vi "B_sweep_versus time_3ch_DR_v2.1.vi"(1 "name or relative path":string="Bsweeps_lockin_sweepVsg1&Vsg2_Vbg9V", 3 "description":string="SA02610M.20130217\ntemp=100mK\n1mVac+350uVdc\nVbg=1V\n", 5 "Stop":bool, 8 "slow scan through zero?":bool, 11 "sec to stablize B":u32=10, 15 "B Start (Oe)":dbl=20000.0, 16 "B End (Oe)":dbl=-20000.0, 17 "B Scan (Oe/sec)":dbl=10.0) -> (0 "Pickering":string="Vbg:27\nV1+:2\nI-:4\nI+:1\nV2-:5\nV2-:28\nV2+:2\nV-:3\n", 10 "Zx 2":cluster{"Y":dbl[], "Y":dbl[]}(graph), 12 "Zx":cluster{"Y":dbl[], "Y":dbl[]}(graph), 13 "T":cluster{"Y":dbl[], "Y":dbl[]}(graph), 18 "Y Channel":cluster{"Y":dbl[], "Y":dbl[]}(graph), 19 "X Channel":cluster{"Y":dbl[], "Y":dbl[]}(graph))   [LabVIEW 2011]
uses:
  SubVI/ITX_Global.vi
  DAQ-lockin-SubVI/Source/Lock-in Globles.vi
panel:
  out "Current field (Oe)":dbl=-19995.404
  in  "Tab Control":T1(tab)
  in  "Lock-in #":u16(ring) items=["Lock-in #1", "Lock-in #2", "Lock-in #3", "Lock-in #4"]
  in  "Lock-in # 3":u16(ring)=2 items=["Lock-in #1", "Lock-in #2", "Lock-in #3", "Lock-in #4"]
  in  "Lock-in # 4":u16(ring)=3 items=["Lock-in #1", "Lock-in #2", "Lock-in #3", "Lock-in #4"]
  in  "Device image":path=path "C:/Experiments/2011-summer Superconductivity-Spin Hall/Device images/SA02610M.20121218.png"
  out "Last Scan Image":T2(plugin-control)
  in  "Initial Rate (Oe/s)":i32=100
  in  "Stop Lockin":bool
  out "X 3":cluster{"Y":dbl[], "Y":dbl[]}(graph)
  out "Y 3":cluster{"Y":dbl[], "Y":dbl[]}(graph)
  out "X 4":cluster{"Y":dbl[], "Y":dbl[]}(graph)
  out "Y4":cluster{"Y":dbl[], "Y":dbl[]}(graph)
  out "Zy":cluster{"Y":dbl[], "Y":dbl[]}(graph)
  out "Zy 2":cluster{"Y":dbl[], "Y":dbl[]}(graph)
  out "T 2":cluster{"Y":dbl[], "Y":dbl[]}[](graph)
  # "yes"
  # "no"
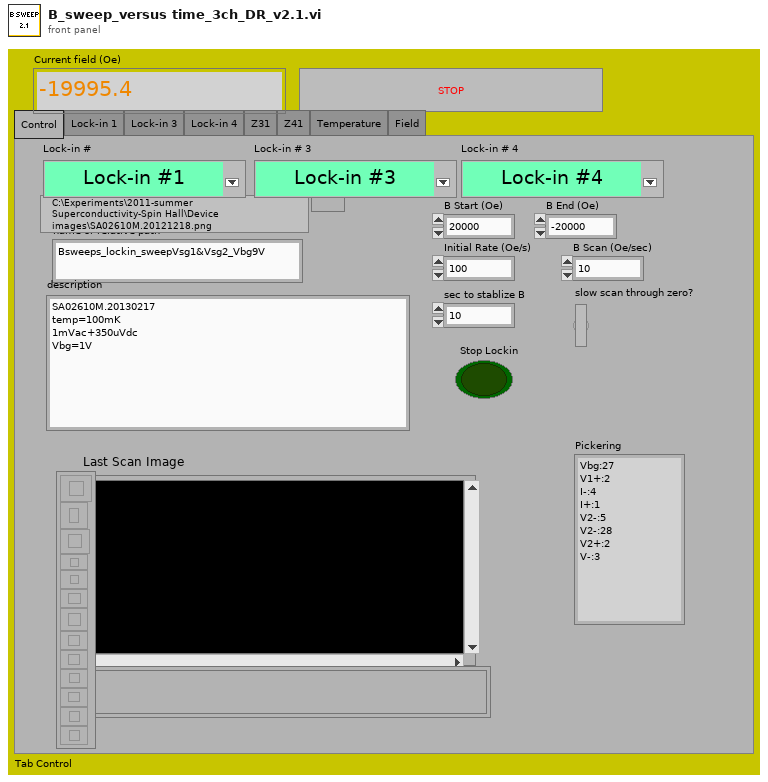
[diagram p1: front panel]
types:
  T1 = enum32{"Control", "Lock-in 1", "Lock-in 3", "Lock-in 4", "Z31", "Z41", "Temperature", "Field"}
  T2 = typedef "IMAQ Image.ctl" = refnum<image>
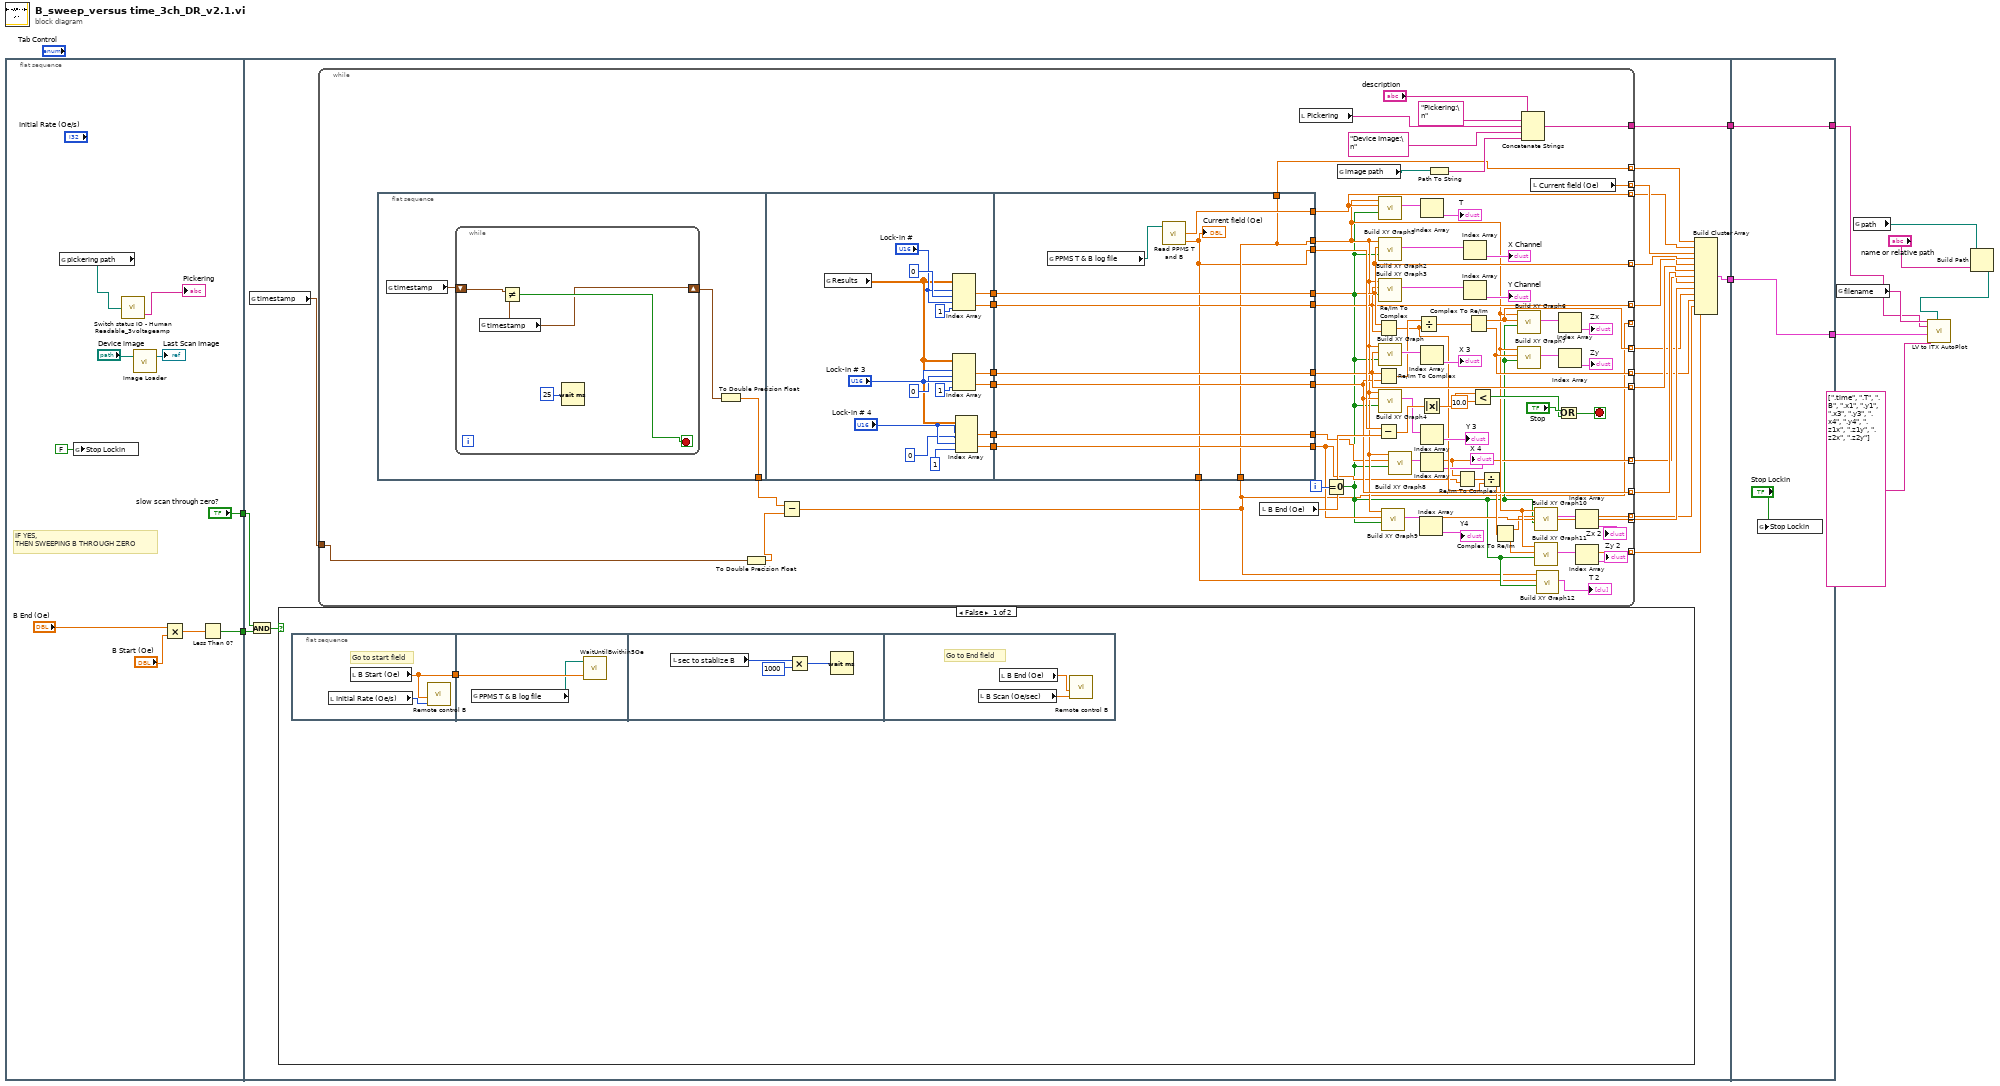
[diagram p0: block diagram]
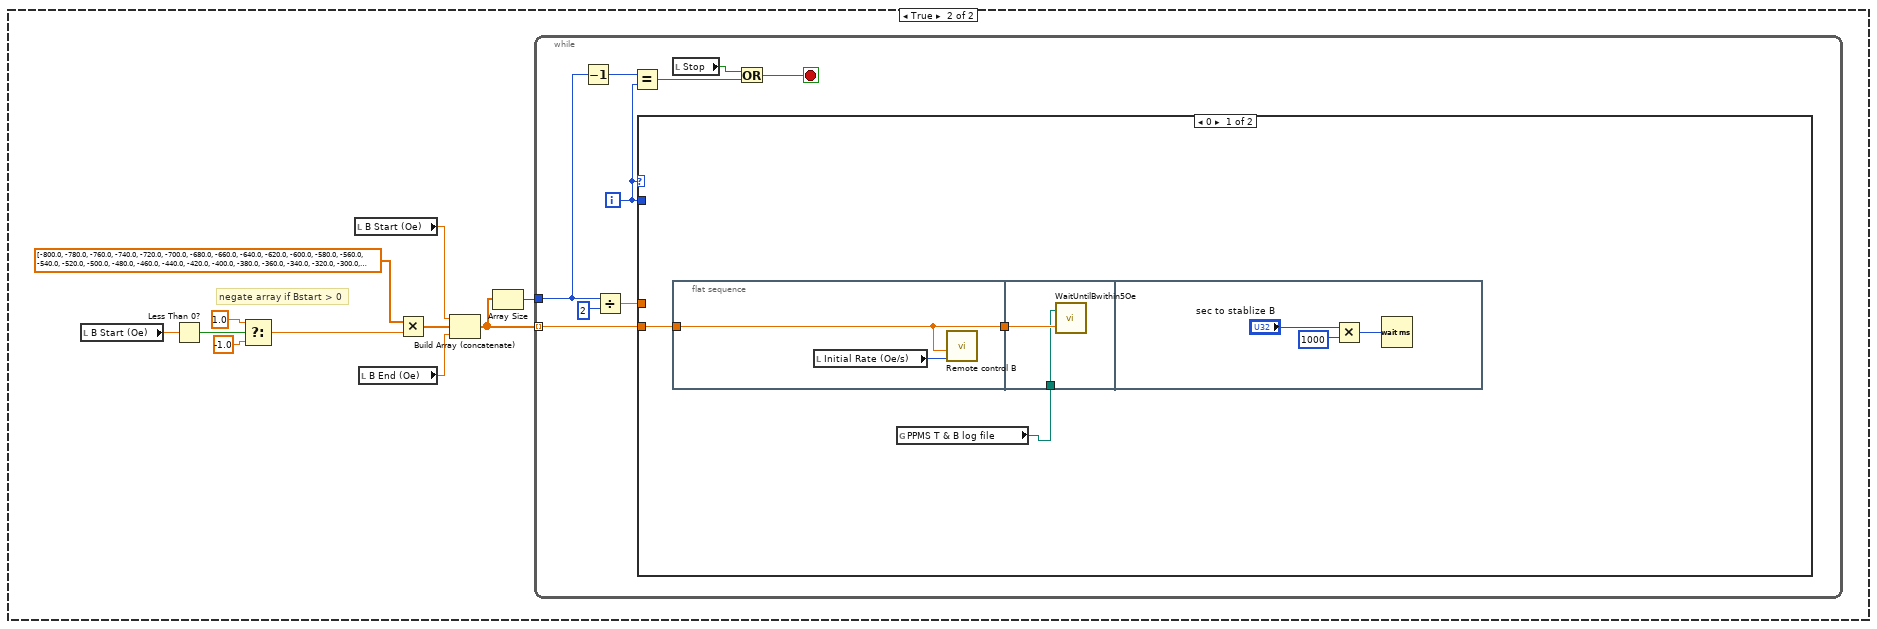
[diagram p2: hidden frame]
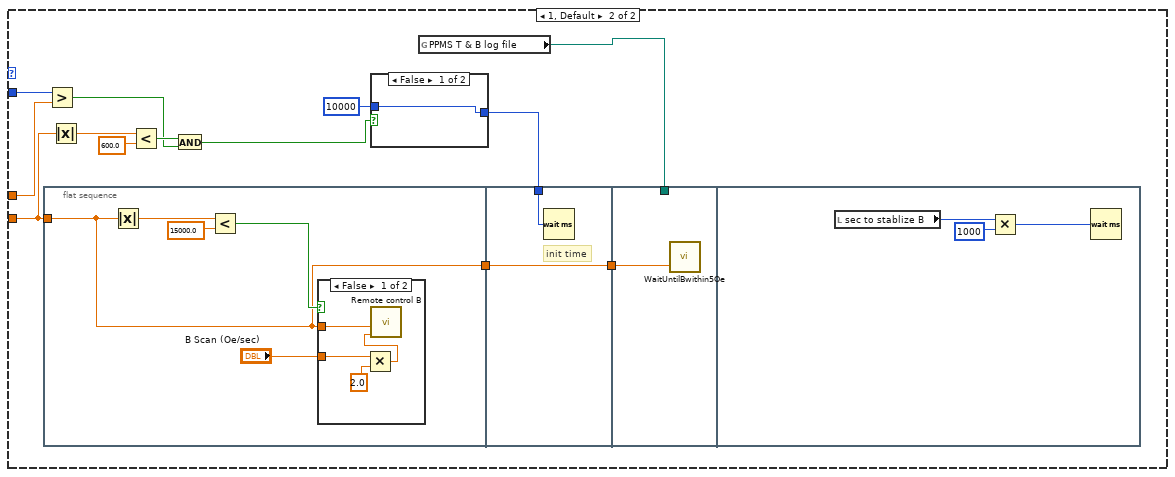
[diagram p3: hidden frame]
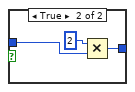
[diagram p4: hidden frame]
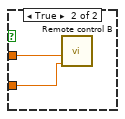
[diagram p5: hidden frame]
diagram:
  n1 = flat-sequence {
    tunnel: [w20] -> w11
    tunnel: ["slow scan through zero?"] -> w10
    tunnel: w11 -> [w40]
    tunnel: w10 -> [w39]
    tunnel: [w37] -> w7
    tunnel: [w24] -> w2
    tunnel: [w220] -> w4
    tunnel: w7 -> [w220]
    tunnel: [w218] -> w3
    tunnel: w2 -> [w218]
    frame #0 {
      # "IF YES,\nTHEN SWEEPING B THROUGH ZERO"
      n2 = global read "ITX_Global.vi" "pickering path"() -> (w13:path)
      n3 = global write "Lock-in Globles.vi" "Stop Lockin"(FALSE ("Stop Lockin")) -> ()
      n4 = call <userlib>:"Switch status IO - Human Readable_3voltageamp.vi"("Switch status"=w13) -> ("String"=→"Pickering":string)  [unwired: 3 in]
      n5 = call "Image Loader.vi"("File Path"="Device image") -> ("Last Scan Image"=→"Last Scan Image":T2)  [unwired: 2 in]
      n6 = Multiply(x="B End (Oe)", y="B Start (Oe)") -> (x*y=w21:dbl)
      n7 = Less Than 0?(x=w21) -> (x < 0?=w20:bool)
    }
    frame #1 {
      n8 = global read "Lock-in Globles.vi" "timestamp"() -> (w22:timestamp)
      n9 = And(x=w39, y=w40) -> (x .and. y?=w38:bool)
      n10 = case shown="False" w38 {
        frame False {
          n11 = flat-sequence {
            tunnel: [w42] -> w41
            tunnel: w41 -> [w45]
            frame #0 {
              # "Go to start field"
              n12 = local read "Initial Rate (Oe/s)"() -> (w43:i32)
              n13 = local read "B Start (Oe)"() -> (w42:dbl)
              n14 = call "Remote control B.vi"("Rate (Oe/s)"=w43, "Field (Oe)"=w42) -> ()  [unwired: 7 in, 1 out]
            }
            frame #1 {
              n15 = global read "ITX_Global.vi" "PPMS T & B log file"() -> (w44:path)
              n16 = call "WaitUntilBwithin5Oe.vi"("Target Field (Oe)"=w45, "PPMS T & B log file"=w44) -> ()  [unwired: 2 in]
            }
            frame #2 {
              n17 = local read "sec to stablize B"() -> (w46:u32)
              n18 = Multiply(x=w46, y=u32 1000) -> (x*y=w47:u32)
              n19 = Wait (ms)(milliseconds to wait=w47) -> ()  [unwired: 1 out]
            }
            frame #3 {
              # "Go to End field"
              n20 = local read "B Scan (Oe/sec)"() -> (w49:dbl)
              n21 = local read "B End (Oe)"() -> (w50:dbl)
              n22 = call "Remote control B.vi"("Rate (Oe/s)"=w49, "Field (Oe)"=w50) -> ()  [unwired: 7 in, 1 out]
            }
          }
        }
        frame True {
          # "negate array if Bstart > 0"
          n23 = local read "B Start (Oe)"() -> (w61:dbl)
          n24 = Less Than 0?(x=w61) -> (x < 0?=w59:bool)
          n25 = Select(t=1.0, s=w59, f=-1.0) -> (s? t:f=w58:dbl)
          n26 = local read "B Start (Oe)"() -> (w53:dbl)
          n27 = local read "B End (Oe)"() -> (w54:dbl)
          n28 = Multiply(x=dbl[] [-800.0, -780.0, -760.0, -740.0, -720.0, -700.0, -680.0, -660.0, -640.0, -620.0, -600.0, -580.0, -560.0, -540.0, -520.0, -500.0, -480.0, -460.0, -440.0, -420.0, -400.0, -380.0, -360.0, -340.0, -320.0, -300.0, -280.0, -260.0, -240.0, -220.0, -200.0, -190.0, -180.0, -170.0, -160.0, -150.0, -140.0, -130.0, -120.0, -110.0, -100.0, -90.0, -80.0, -70.0, -60.0, -50.0, -40.0, -30.0, -20.0, -10.0, 0.0, 10.0, 20.0, 30.0, 40.0, 50.0, 60.0, 70.0, 80.0, 90.0, 100.0, 110.0, 120.0, 130.0, 140.0, 150.0, 160.0, 170.0, 180.0, 190.0, 200.0, 220.0, 240.0, 260.0, 280.0, 300.0, 320.0, 340.0, 360.0, 380.0, 400.0, 420.0, 440.0, 460.0, 480.0, 500.0, 520.0, 540.0, 560.0, 580.0, 600.0, 620.0, 640.0, 660.0, 680.0, 700.0, 720.0, 740.0, 760.0, 780.0, 800.0], y=w58) -> (x*y=w55:dbl[])
          n29 = Build Array (concatenate)(w53, w55, w54) -> (w52:dbl[])
          n30 = Array Size(array=w52) -> (size(s)=w51:i32)
          n31 = while {
            tunnel: w52 -> [w70] mode=indexing
            tunnel: w51 -> [w65]
            i -> [w62]
            stop <- w66 stop-if-true
            n32 = Decrement(x=w65) -> (x-1=w69:i32)
            n33 = Divide(x=w65, y=2) -> (x/y=w63:dbl)
            n34 = Equal?(x=w69, y=w62) -> (x = y?=w68:bool)
            n35 = case shown="0" w62 {
              tunnel: w70 -> [w72 w91]
              tunnel: w63 -> [_ w87]
              tunnel: w62 -> [_ w86]
              frame 0 {
                n36 = flat-sequence {
                  tunnel: w72 -> [w75]
                  tunnel: [w75] -> w73
                  tunnel: w71 -> [w76]
                  tunnel: w73 -> [w77]
                  frame #0 {
                    n37 = local read "Initial Rate (Oe/s)"() -> (w74:i32)
                    n38 = call "Remote control B.vi"("Rate (Oe/s)"=w74, "Field (Oe)"=w75) -> ()  [unwired: 7 in, 1 out]
                  }
                  frame #1 {
                    n39 = call "WaitUntilBwithin5Oe.vi"("Target Field (Oe)"=w77, "PPMS T & B log file"=w76) -> ()  [unwired: 2 in]
                  }
                  frame #2 {
                    n40 = Multiply(x="sec to stablize B", y=u32 1000) -> (x*y=w79:u32)
                    n41 = Wait (ms)(milliseconds to wait=w79) -> ()  [unwired: 1 out]
                  }
                }
                n42 = global read "ITX_Global.vi" "PPMS T & B log file"() -> (w71:path)
              }
              frame 1, Default {
                n43 = flat-sequence {
                  tunnel: w91 -> [w99]
                  tunnel: [w99] -> w93
                  tunnel: w93 -> [w110]
                  tunnel: [w110] -> w92
                  tunnel: w82 -> [w109]
                  tunnel: w81 -> [_]
                  tunnel: w92 -> [w111]
                  frame #0 {
                    n44 = Absolute Value(x=w99) -> (abs(x)=w98:dbl)
                    n45 = Less?(x=w98, y=15000.0) -> (x < y?=w100:bool)
                    n46 = case shown="False" w100 {
                      tunnel: w99 -> [w106 w108]
                      tunnel: "B Scan (Oe/sec)" -> [w105 w107]
                      frame False {
                        n47 = Multiply(x=w105, y=2.0) -> (x*y=w103:dbl)
                        n48 = call "Remote control B.vi"("Rate (Oe/s)"=w103, "Field (Oe)"=w106) -> ()  [unwired: 7 in, 1 out]
                      }
                      frame True {
                        n49 = call "Remote control B.vi"("Rate (Oe/s)"=w107, "Field (Oe)"=w108) -> ()  [unwired: 7 in, 1 out]
                      }
                    }
                  }
                  frame #1 {
                    # "init time"
                    n50 = Wait (ms)(milliseconds to wait=w109) -> ()  [unwired: 1 out]
                  }
                  frame #2 {
                    n51 = call "WaitUntilBwithin5Oe.vi"("Target Field (Oe)"=w111) -> ()  [unwired: 3 in]
                  }
                  frame #3 {
                    n52 = local read "sec to stablize B"() -> (w112:u32)
                    n53 = Multiply(x=w112, y=u32 1000) -> (x*y=w113:u32)
                    n54 = Wait (ms)(milliseconds to wait=w113) -> ()  [unwired: 1 out]
                  }
                }
                n55 = Greater?(x=w86, y=w87) -> (0:w85:bool)
                n56 = Absolute Value(x=w91) -> (abs(x)=w88:dbl)
                n57 = Less?(x=w88, y=600.0) -> (x < y?=w89:bool)
                n58 = And(x=w89, y=w85) -> (x .and. y?=w84:bool)
                n59 = case shown="False" w84 {
                  tunnel: u32 10000 ("y") -> [w94 w97]
                  tunnel: [w94 w95] -> w82
                  frame False {
                  }
                  frame True {
                    n60 = Multiply(x=u32 2, y=w97) -> (x*y=w95:u32)
                  }
                }
                n61 = global read "ITX_Global.vi" "PPMS T & B log file"() -> (w81:path)
              }
            }
            n62 = local read "Stop"() -> (w67:bool)
            n63 = Or(x=w67, y=w68) -> (x .or. y?=w66:bool)
          }
        }
      }
      n64 = while {
        tunnel: [w115] -> _ mode=indexing
        tunnel: [w155] -> w35 mode=indexing
        tunnel: [w154] -> w36 mode=indexing
        tunnel: [w153] -> w34 mode=indexing
        tunnel: [w152] -> w32 mode=indexing
        tunnel: [w151] -> w33 mode=indexing
        tunnel: [w150] -> w31 mode=indexing
        tunnel: [w149] -> w28 mode=indexing
        tunnel: [w148] -> w27 mode=indexing
        tunnel: [w127] -> w37
        tunnel: [w126] -> w30 mode=indexing
        tunnel: [w125] -> w29 mode=indexing
        tunnel: [w124] -> w26 mode=indexing
        tunnel: [w123] -> w25 mode=indexing
        tunnel: [w119] -> w23 mode=indexing
        tunnel: w22 -> [w118]
        i -> [w184]
        stop <- w177 stop-if-true
        n65 = flat-sequence {
          tunnel: [w187] -> w117
          tunnel: [w204] -> w159
          tunnel: [w203] -> w158
          tunnel: [w199] -> w157
          tunnel: [w198] -> w156
          tunnel: [w193] -> w147
          tunnel: [w192] -> w146
          tunnel: [w209] -> w136
          tunnel: [w208] -> w167
          tunnel: w159 -> [w217]
          tunnel: [w217] -> w151
          tunnel: w158 -> [w216]
          tunnel: [w216] -> w153
          tunnel: [w215] -> w152
          tunnel: w157 -> [w215]
          tunnel: w156 -> [w214]
          tunnel: [w214] -> w150
          tunnel: [w213] -> w155
          tunnel: [w212] -> w126
          tunnel: w147 -> [w212]
          tunnel: [w211] -> w125
          tunnel: w146 -> [w211]
          tunnel: w115 -> [w209]
          tunnel: [w208] -> w121
          tunnel: [w209] -> w119
          frame #0 {
            n66 = global read "Lock-in Globles.vi" "timestamp"() -> (w186:timestamp)
            n67 = while {
              shift-right: [w189] -> w185
              shift-left: w186 -> [w191]
              stop <- w190 stop-if-true
              n68 = global read "Lock-in Globles.vi" "timestamp"() -> (w189:timestamp)
              n69 = Not Equal?(x=w191, y=w189) -> (x != y?=w190:bool)
              n70 = Wait (ms)(milliseconds to wait=u32 25) -> ()  [unwired: 1 out]
            }
            n71 = To Double Precision Float(number=w185) -> (double precision float=w187:dbl)
          }
          frame #1 {
            n72 = global read "Lock-in Globles.vi" "Results"() -> (w194:dbl[][])
            n73 = Index Array(array=w194, index (row) #1="Lock-in #", index (col) #1=0 ("disabled index (col)"), index (row) #2="Lock-in #", index (col) #2=1 ("disabled index (col)")) -> (element #1=w203:dbl, element #2=w204:dbl)
            n74 = Index Array(array=w194, index (row) #1="Lock-in # 3", index (col) #1=0 ("disabled index (col)"), index (row) #2="Lock-in # 3", index (col) #2=1 ("disabled index (col)")) -> (element #1=w199:dbl, element #2=w198:dbl)
            n75 = Index Array(array=w194, index (row) #1="Lock-in # 4", index (col) #1=0 ("disabled index (col)"), index (row) #2="Lock-in # 4", index (col) #2=1 ("disabled index (col)")) -> (element #1=w193:dbl, element #2=w192:dbl)
          }
          frame #2 {
            n76 = global read "ITX_Global.vi" "PPMS T & B log file"() -> (w210:path)
            n77 = call "Read PPMS T and B.vi"("file (use dialog)"=w210) -> ("Field"=w208:dbl, "Temperature"=w213:dbl)  [unwired: 2 in, 1 out]
            "Current field (Oe)" <- w208
          }
        }
        n78 = To Double Precision Float(number=w118) -> (double precision float=w116:dbl)
        n79 = Subtract(x=w117, y=w116) -> (x-y=w115:dbl)
        n80 = local read "B End (Oe)"() -> (w168:dbl)
        n81 = local read "Pickering"() -> (w129:string)
        n82 = Equal To 0?(x=w184) -> (x = 0?=w122:bool)
        n83 = global read "ITX_Global.vi" "image path"() -> (w128:path)
        n84 = Re/Im To Complex(1:w151, 2:w153) -> (0:w144:cdb)
        n85 = Re/Im To Complex(1:w150, 2:w152) -> (0:w172:cdb)
        n86 = Subtract(x=w167, y=w168) -> (x-y=w182:dbl)
        n87 = call "Build XY Graph5"("Reset"=w122, "Y Input"=w155, "X Input"=w136) -> ("XY Graph"=w173:cluster{"Y":dbl[], "Y":dbl[]}[])  [unwired: 2 in, 6 out]
        n88 = call "Build XY Graph2"("Reset"=w122, "Y Input"=w153, "X Input"=w136) -> ("XY Graph"=w178:cluster{"Y":dbl[], "Y":dbl[]}[])  [unwired: 2 in, 6 out]
        n89 = call "Build XY Graph3"("Reset"=w122, "Y Input"=w151, "X Input"=w136) -> ("XY Graph"=w179:cluster{"Y":dbl[], "Y":dbl[]}[])  [unwired: 2 in, 6 out]
        n90 = call "Build XY Graph"("Reset"=w122, "Y Input"=w152, "X Input"=w136) -> ("XY Graph"=w175:cluster{"Y":dbl[], "Y":dbl[]}[])  [unwired: 2 in, 6 out]
        n91 = call "Build XY Graph4"("Reset"=w122, "Y Input"=w150, "X Input"=w136) -> ("XY Graph"=w174:cluster{"Y":dbl[], "Y":dbl[]}[])  [unwired: 2 in, 6 out]
        n92 = call "Build XY Graph9"("Reset"=w122, "Y Input"=w125, "X Input"=w136) -> ("XY Graph"=w140:cluster{"Y":dbl[], "Y":dbl[]}[])  [unwired: 2 in, 6 out]
        n93 = call "Build XY Graph8"("Reset"=w122, "Y Input"=w126, "X Input"=w136) -> ("XY Graph"=w142:cluster{"Y":dbl[], "Y":dbl[]}[])  [unwired: 2 in, 6 out]
        n94 = Divide(x=w172, y=w144) -> (x/y=w171:cdb)
        n95 = Index Array(array=w140) -> (element=→"Y4":cluster{"Y":dbl[], "Y":dbl[]})  [unwired: 1 in]
        n96 = Index Array(array=w173) -> (element=→"T":cluster{"Y":dbl[], "Y":dbl[]})  [unwired: 1 in]
        n97 = Index Array(array=w175) -> (element=→"X 3":cluster{"Y":dbl[], "Y":dbl[]})  [unwired: 1 in]
        n98 = Absolute Value(x=w182) -> (abs(x)=w181:dbl)
        n99 = Index Array(array=w174) -> (element=→"Y 3":cluster{"Y":dbl[], "Y":dbl[]})  [unwired: 1 in]
        n100 = Index Array(array=w142) -> (element=→"X 4":cluster{"Y":dbl[], "Y":dbl[]})  [unwired: 1 in]
        n101 = Path To String(path=w128) -> (string=w130:string)
        n102 = Re/Im To Complex(1:w125, 2:w126) -> (0:w145:cdb)
        n103 = Index Array(array=w178) -> (element=→"X Channel":cluster{"Y":dbl[], "Y":dbl[]})  [unwired: 1 in]
        n104 = Index Array(array=w179) -> (element=→"Y Channel":cluster{"Y":dbl[], "Y":dbl[]})  [unwired: 1 in]
        n105 = Complex To Re/Im(x + iy=w171) -> (x=w149:dbl, y=w148:dbl)
        n106 = Less?(x=w181, y=10.0) -> (x < y?=w176:bool)
        n107 = Divide(x=w145, y=w144) -> (x/y=w143:cdb)
        n108 = Complex To Re/Im(x + iy=w143) -> (x=w124:dbl, y=w123:dbl)
        n109 = call "Build XY Graph6"("Reset"=w122, "Y Input"=w149, "X Input"=w136) -> ("XY Graph"=w170:cluster{"Y":dbl[], "Y":dbl[]}[])  [unwired: 2 in, 6 out]
        n110 = call "Build XY Graph7"("Reset"=w122, "Y Input"=w148, "X Input"=w136) -> ("XY Graph"=w169:cluster{"Y":dbl[], "Y":dbl[]}[])  [unwired: 2 in, 6 out]
        n111 = Concatenate Strings("description", "Pickering:\n" ("string"), w129, "Device Image:\n" ("string"), w130) -> (w127:string)
        n112 = local read "Current field (Oe)"() -> (w154:dbl)
        n113 = call "Build XY Graph10"("Reset"=w122, "Y Input"=w124, "X Input"=w136) -> ("XY Graph"=w137:cluster{"Y":dbl[], "Y":dbl[]}[])  [unwired: 2 in, 6 out]
        n114 = call "Build XY Graph11"("Reset"=w122, "Y Input"=w123, "X Input"=w136) -> ("XY Graph"=w138:cluster{"Y":dbl[], "Y":dbl[]}[])  [unwired: 2 in, 6 out]
        n115 = call "Build XY Graph12"("Reset"=w122, "Y Input"=w121, "X Input"=w115) -> ("XY Graph"=→"T 2":cluster{"Y":dbl[], "Y":dbl[]}[])  [unwired: 2 in, 6 out]
        n116 = Or(x="Stop", y=w176) -> (x .or. y?=w177:bool)
        n117 = Index Array(array=w170) -> (element=→"Zx":cluster{"Y":dbl[], "Y":dbl[]})  [unwired: 1 in]
        n118 = Index Array(array=w169) -> (element=→"Zy":cluster{"Y":dbl[], "Y":dbl[]})  [unwired: 1 in]
        n119 = Index Array(array=w137) -> (element=→"Zx 2":cluster{"Y":dbl[], "Y":dbl[]})  [unwired: 1 in]
        n120 = Index Array(array=w138) -> (element=→"Zy 2":cluster{"Y":dbl[], "Y":dbl[]})  [unwired: 1 in]
      }
      n121 = Build Cluster Array(w23, w35, w36, w34, w33, w32, w31, w30, w29, w28, w27, w26, w25) -> (w24:cluster{dbl[]}[])
    }
    frame #2 {
      n122 = global write "Lock-in Globles.vi" "Stop Lockin"("Stop Lockin") -> ()
    }
  }
  n123 = global read "ITX_Global.vi" "filename"() -> (w5:string)
  n124 = global read "ITX_Global.vi" "path"() -> (w9:path)
  n125 = Build Path(base path=w9, name or relative path="name or relative path") -> (appended path=w6:path)
  n126 = call <userlib>:"LV to ITX AutoPlot.vi"("filename"=w5, "path"=w6, "Notes"=w4, "Data"=w3, "wavenames (.Vx, etc)"=string[] [".time", ".T", ".B", ".x1", ".y1", ".x3", ".y3", ".x4", ".y4", ".z1x", ".z1y", ".z2x", ".z2y"]) -> ()  [unwired: 10 in, 1 out]
